vi "9205_Update Ring Controls.vi"(5 "SelectedChannels":i32[](array[numeric]), 7 "ChannelConfig":u8[](array[numeric]), 9 "SupportedModes":string[][](array[string])) -> (6 "Strings out":string[](array[string]), 8 "Disabled Items out":i32[](array[numeric]), 10 "Value out":u8, 15 "Visible out":bool)   [LabVIEW 2019, in "Modules.lvlib" / "9205.lvclass"]
uses:
  9205.lvclass
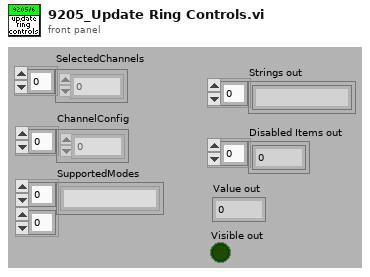
[diagram p1: front panel]
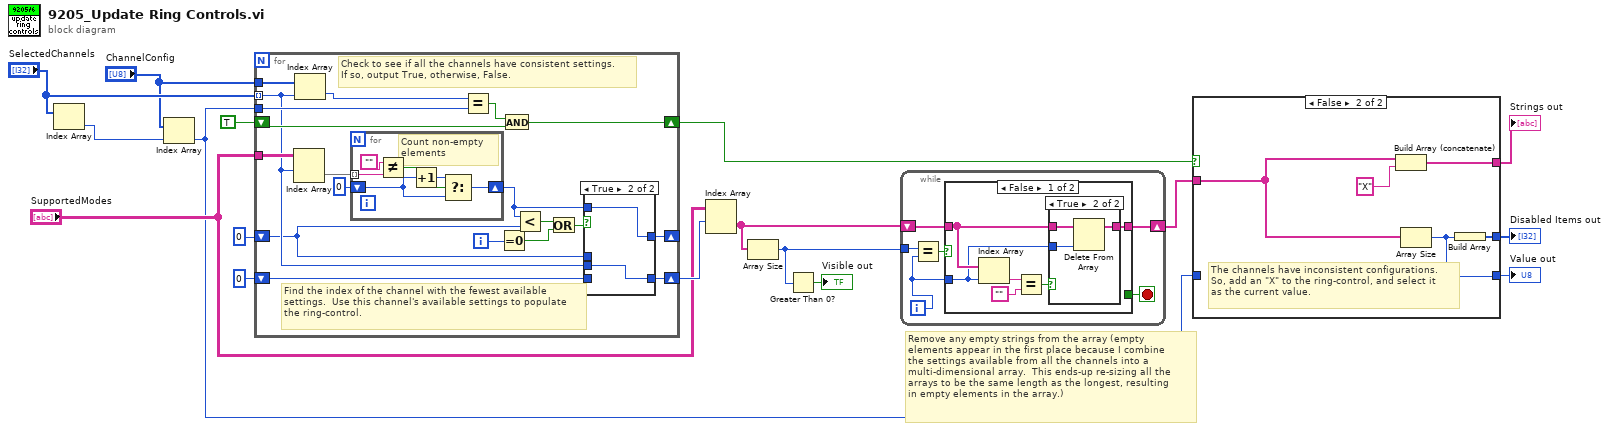
[diagram p0: block diagram]
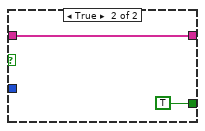
[diagram p3: hidden frame]
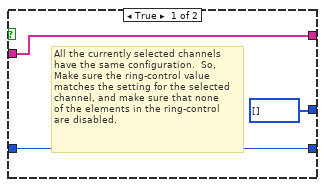
[diagram p5: hidden frame]
diagram:
  # "Remove any empty strings from the array (empty\nelements appear in the first place because I combine\nthe settings available from all the channels into a \nmulti-dimensional array.  This ends-up re-sizing all the\narrays to be the same length as the longest, resulting\nin empty elements in the array.)"
  n1 = Index Array(array="SelectedChannels") -> (element=w11:i32)  [unwired: 1 in]
  n2 = Index Array(array="ChannelConfig", index=w11) -> (element=w5:u8)
  n3 = for {
    tunnel: "SelectedChannels" -> [w28] mode=indexing
    tunnel: w5 -> [w35]
    shift-right: [w33] -> w10
    shift-left: TRUE -> [w32]
    tunnel: "ChannelConfig" -> [w31]
    tunnel: "SupportedModes" -> [w30]
    shift-right: [w29] -> _
    shift-left: 0 -> [w22]
    shift-right: [w27] -> w7
    shift-left: 0 ("Numeric") -> [w21]
    i -> [w24]
    # "Find the index of the channel with the fewest available\nsettings.  Use this channel's available settings to populate\nthe ring-control."
    # "Check to see if all the channels have consistent settings.\nIf so, output True, otherwise, False."
    n4 = Index Array(array=w30, index (row)=w28) -> (element=w20:string[])  [unwired: 1 in]
    n5 = Index Array(array=w31, index=w28) -> (element=w36:u8)
    n6 = for {
      shift-right: [w37] -> w18
      shift-left: 0 -> [w38]
      tunnel: w20 -> [w42] mode=indexing
      # "Count non-empty\nelements"
      n7 = Not Equal?(x="", y=w42) -> (x != y?=w40:bool)
      n8 = Increment(x=w38) -> (x+1=w39:i32)
      n9 = Select(t=w39, s=w40, f=w38) -> (s? t:f=w37:i32)
    }
    n10 = Equal?(x=w36, y=w35) -> (x = y?=w34:bool)
    n11 = Equal To 0?(x=w24) -> (x = 0?=w23:bool)
    n12 = And(x=w34, y=w32) -> (x .and. y?=w33:bool)
    n13 = Less?(x=w18, y=w22) -> (x < y?=w26:bool)
    n14 = Or(x=w26, y=w23) -> (x .or. y?=w25:bool)
    n15 = case shown="True" w25 {
      tunnel: w18 -> [_ w46]
      tunnel: [w44 w46] -> w29
      tunnel: w28 -> [_ w45]
      tunnel: [w43 w45] -> w27
      tunnel: w22 -> [w44 _]
      tunnel: w21 -> [w43 _]
      frame False {
      }
      frame True {
      }
    }
  }
  n16 = Index Array(array="SupportedModes", index (row)=w7) -> (element=w4:string[])  [unwired: 1 in]
  n17 = Array Size(array=w4) -> (size(s)=w2:i32)
  n18 = Greater Than 0?(x=w2) -> (x > 0?=→"Visible out":bool)
  n19 = while {
    shift-right: [w48] -> w3
    shift-left: w4 -> [w49]
    tunnel: w2 -> [w51]
    i -> [w47]
    stop <- w50 stop-if-true
    n20 = Equal?(x=w51, y=w47) -> (x = y?=w52:bool)
    n21 = case shown="False" w52 {
      tunnel: [_ TRUE] -> w50
      tunnel: [w53 w63] -> w48
      tunnel: w49 -> [w55 w63]
      tunnel: w47 -> [w54 _]
      frame False {
        n22 = Index Array(array=w55, index=w54) -> (element=w58:string)
        n23 = Equal?(x=w58, y="") -> (x = y?=w56:bool)
        n24 = case shown="True" w56 {
          tunnel: w55 -> [w59 w62]
          tunnel: w54 -> [_ w61]
          tunnel: [w59 w60] -> w53
          frame False {
          }
          frame True {
            n25 = Delete From Array(array=w62, index=w61) -> (array with subset deleted=w60:string[])  [unwired: 1 in, 1 out]
          }
        }
      }
      frame True {
      }
    }
  }
  n26 = case shown="False" w10 {
    tunnel: w3 -> [w67 w72]
    tunnel: [w67 w71] -> w15
    tunnel: [i32[] [] w70] -> w16
    tunnel: w5 -> [w66 _]
    tunnel: [w66 w69] -> w17
    frame True {
      # "All the currently selected channels\nhave the same configuration.  So,\nMake sure the ring-control value\nmatches the setting for the selected\nchannel, and make sure that none\nof the elements in the ring-control\nare disabled."
    }
    frame False {
      # "The channels have inconsistent configurations.\nSo, add an \"X\" to the ring-control, and select it\nas the current value."
      n27 = Build Array (concatenate)(w72, "X" ("String")) -> (w71:string[])
      n28 = Array Size(array=w72) -> (size(s)=w69:i32)
      n29 = Build Array(w69) -> (w70:i32[])
    }
  }
  "Value out" <- w17
  "Disabled Items out" <- w16
  "Strings out" <- w15
